vi "_PC_NS_SubVI_UpperTime.vi"(0 "Init Time":i32=500, 1 "Init? (F)":bool, 2 "Update (T)":bool=TRUE) -> (5 "UpdateTime":i32)   [LabVIEW 2018]
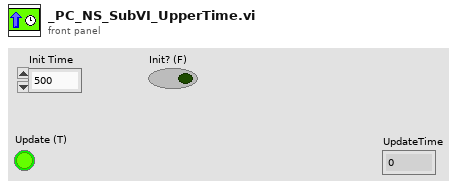
[diagram p1: front panel]
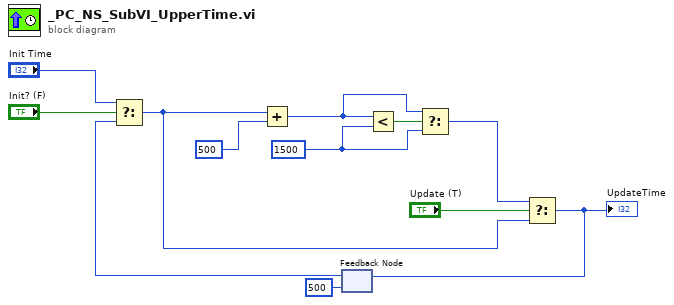
[diagram p0: block diagram]
diagram:
  w9 = 1500 ("y")
  n1 = feedback #1(500 ("Init Time")) -> (w3:i32)
  n2 = Select(t="Init Time", s="Init? (F)", f=w3) -> (s? t:f=w2:i32)
  n3 = Add(x=w2, y=500) -> (x+y=w10:i32)
  n4 = Less?(x=w10, y=w9) -> (x < y?=w11:bool)
  n5 = Select(t=w10, s=w11, f=w9) -> (s? t:f=w7:i32)
  n6 = Select(t=w7, s="Update (T)", f=w2) -> (s? t:f=w4:i32)
  "UpdateTime" <- w4
  n7 = feedback-in #1(w4) -> ()
